vi "At_Goal_Pos.vi"(9 "max Difference":i32, 11 "array":i32[](array[numeric])) -> (2 "At Pos?":bool)   [LabVIEW 2015]
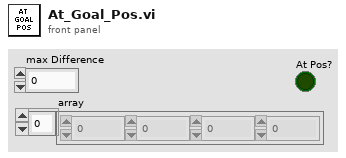
[diagram p1: front panel]
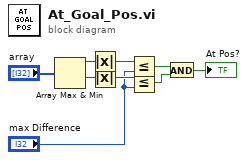
[diagram p0: block diagram]
diagram:
  n1 = Array Max & Min(array="array") -> (max value=w9:i32, min value=w8:i32)  [unwired: 2 out]
  n2 = Absolute Value(x=w9) -> (abs(x)=w6:i32)
  n3 = Absolute Value(x=w8) -> (abs(x)=w5:i32)
  n4 = Less Or Equal?(x=w6, y="max Difference") -> (x <= y?=w4:bool)
  n5 = Less Or Equal?(x=w5, y="max Difference") -> (x <= y?=w3:bool)
  n6 = And(x=w4, y=w3) -> (x .and. y?=→"At Pos?":bool)
